vi "FM Voice Receiver - FIR.vi"() -> ()   [LabVIEW 2013]
uses:
  <vilib>/sound2/lvsound2.llb/Sound Output Write (DBL).vi
  <instrlib>/niUSRP/niUSRP Fetch Rx Data (CDB WDT).vi
  <vilib>/Analysis/3filter.llb/FIR Filter (DBL).vi
  <vilib>/Analysis/2dsp.llb/Rational Resample (single channel, DBL).vi
  <vilib>/express/express analysis/Spectral/Block/exnSpectralBlock spectral measurements RMS poly.vi
  <vilib>/express/express analysis/Spectral/Block/exnSpectralBlock spectral measurements RMS WFM.vi
  <vilib>/express/express analysis/Spectral/XNode/ExpressSpectralMeasurementsBlockNode.xnode
  <vilib>/Analysis/NI_AALPro.lvlib
  <vilib>/Analysis/NI_AALBase.lvlib
panel:
  out "File Error Out":errorcluster
  in  "Sound Format":T1={"sample rate (S/s)"=44100.0, "number of channels"=1.0, "bits per sample"=16.0}
  out "Spectrum (FFT)":cluster{"f0":dbl, "df":dbl, "magnitude":dbl[]}(graph)
  out "Waveform":waveform(dbl)(graph)
  out "Constellation":cluster{dbl[], dbl[]}(graph)
  out "USRP Error Out":errorcluster
  out "Coerced Gain":dbl format="%#_6f"
  out "Coerced Carrier Freq.":dbl=2400010000.007024 format="%#_6p"
  out "Coerced IQ Rate":dbl=200000.0 format="%#_6p"
  in  "Stop":bool
  in  "Active Antenna":string="RX2"
  in  "Gain":dbl format="%#_6f"
  in  "Carrier Frequency":dbl=1200000000.0 format="%#_6p"
  in  "IQ Rate":dbl=200000.0 format="%#_6p"
  in  "Device Address":refnum<k15>="192.168.10.2"
  in  "Number of Samples":i32=44100
  # "FM Receiver"
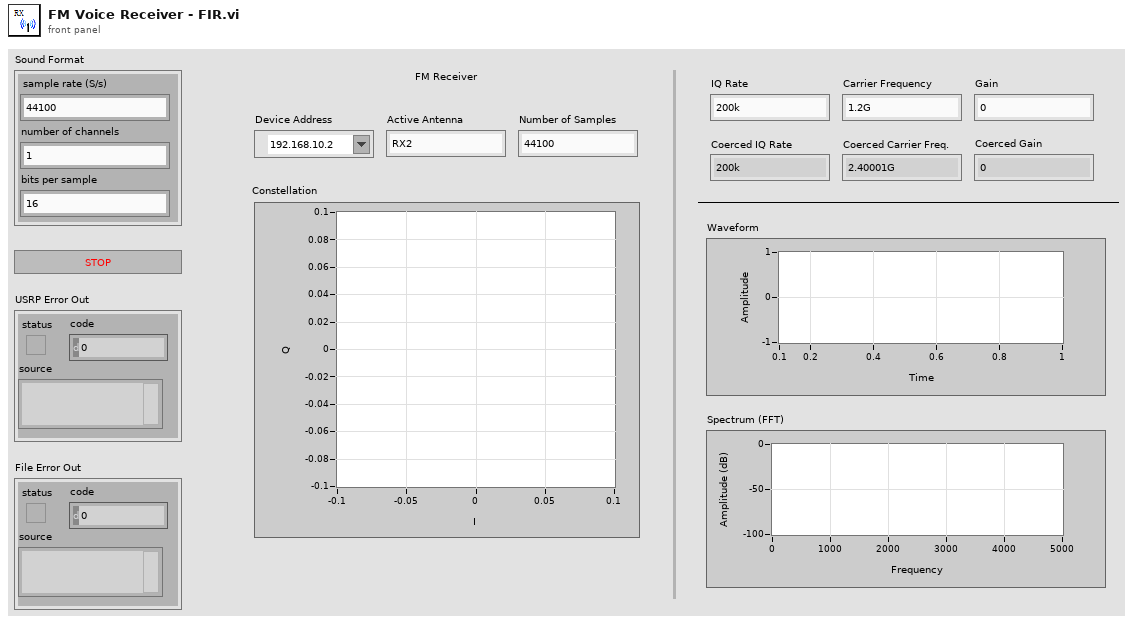
[diagram p1: front panel]
types:
  T1 = cluster{"sample rate (S/s)":dbl, "number of channels":dbl, "bits per sample":dbl}
  T2 = typedef "Sound Output Task ID.ctl" = u32
  T3 = cluster{"averaging mode":u16, "weighting mode":u16, "number of averages":u32}
  T4 = cluster{"dB On (F)":bool, "unwrap phase (F)":bool, "convert to degree (F)":bool}
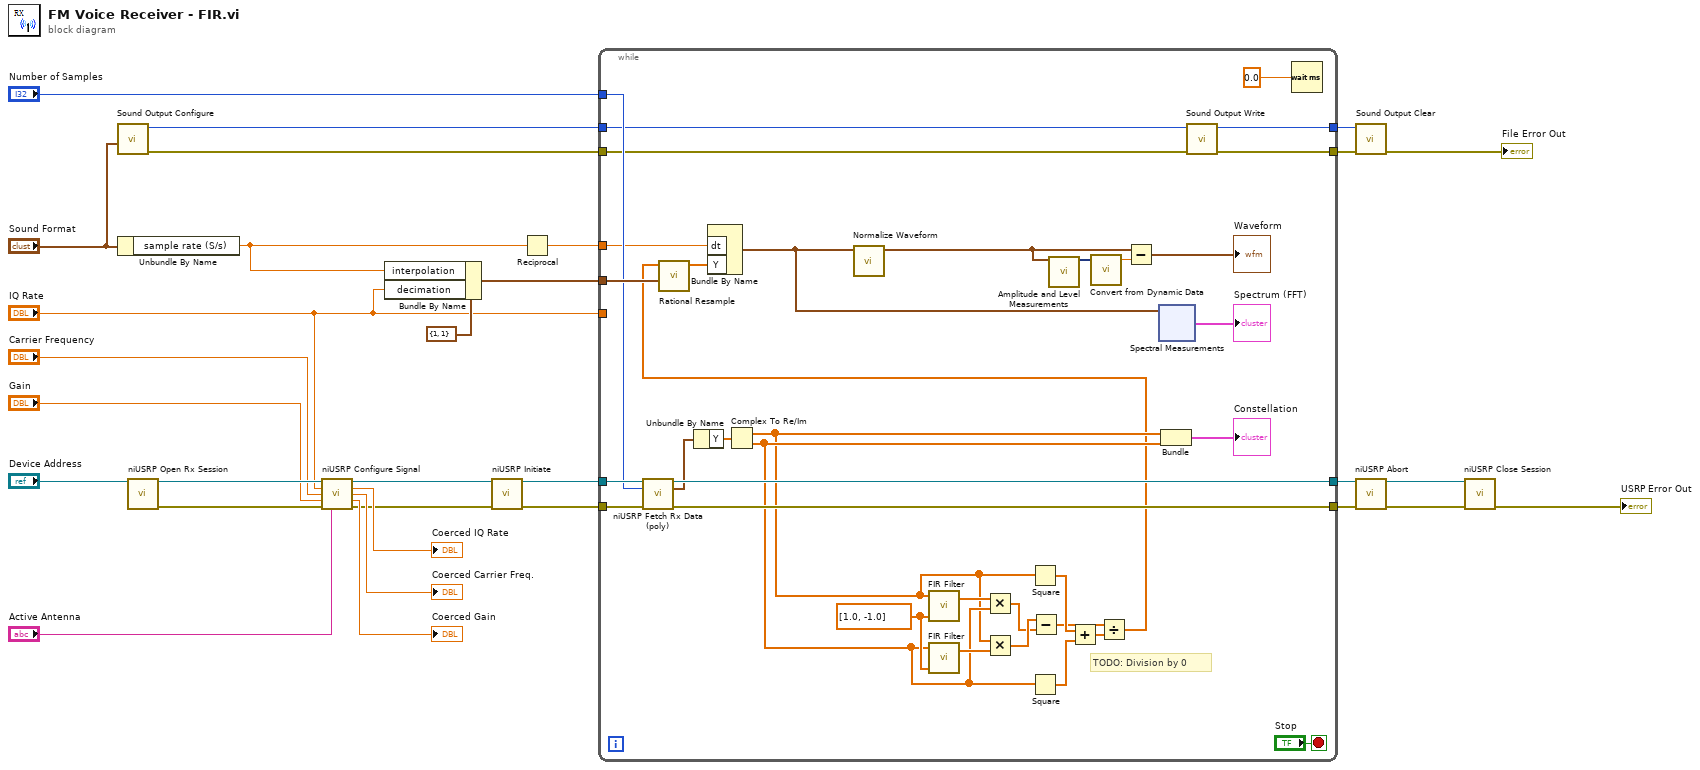
[diagram p0: block diagram]
diagram:
  n1 = call <vilib>:"Sound Output Configure.vi"("sound format"="Sound Format") -> ("error out"=w4:errorcluster, "task ID"=w5:T2)  [unwired: 9 in]
  n2 = Unbundle By Name("Sound Format") -> ("sample rate (S/s)"=w12:dbl)
  n3 = call <instrlib>:"niUSRP Open Rx Session.vi"("device names"="Device Address") -> ("session handle out"=w30:refnum<k15>, "error out"=w29:errorcluster)  [unwired: 13 in]
  n4 = call <instrlib>:"niUSRP Configure Signal.vi"("session handle"=w30, "IQ rate"="IQ Rate", "carrier frequency"="Carrier Frequency", "gain"="Gain", "error in (no error)"=w29, "active antenna"="Active Antenna") -> ("session handle out"=w16:refnum<k15>, "coerced IQ rate"=→"Coerced IQ Rate":dbl, "coerced carrier frequency"=→"Coerced Carrier Freq.":dbl, "coerced gain"=→"Coerced Gain":dbl, "error out"=w14:errorcluster)  [unwired: 5 in]
  n5 = Bundle By Name(cluster=cluster{"decimation":i32, "interpolation":i32} {"decimation"=1, "interpolation"=1}, "interpolation"=w12, "decimation"="IQ Rate") -> (w24:cluster{"decimation":i32, "interpolation":i32})
  n6 = call <instrlib>:"niUSRP Initiate.vi"("session handle"=w16, "error in (no error)"=w14) -> ("session handle out"=w15:refnum<k15>, "error out"=w13:errorcluster)  [unwired: 12 in]
  n7 = Reciprocal(x=w12) -> (1/x=w7:dbl)
  n8 = while {
    tunnel: w15 -> [w65]
    tunnel: [w63] -> w11
    tunnel: [w62] -> w10
    tunnel: w13 -> [w61]
    tunnel: "Number of Samples" -> [w57]
    tunnel: w24 -> [w60]
    tunnel: "IQ Rate" -> [_]
    tunnel: w7 -> [w53]
    tunnel: w5 -> [w52]
    tunnel: w4 -> [w51]
    tunnel: [w50] -> w3
    tunnel: [w49] -> w2
    stop <- "Stop" stop-if-true
    w38 = dbl[] [1.0, -1.0]
    # "TODO: Division by 0"
    n9 = call-poly <instrlib>:"niUSRP Fetch Rx Data (poly).vi"("session handle"=w65, "number of samples"=w57, "error in (no error)"=w61) -> ("session handle out"=w63:refnum<k15>, "data"=w43:waveform(cdb), "error out"=w62:errorcluster)  [unwired: 9 in, 1 out]
    n10 = Unbundle By Name(w43) -> ("Y"=w56:cdb[])
    n11 = Complex To Re/Im(x + iy=w56) -> (x=w36:dbl[], y=w37:dbl[])
    n12 = call-poly <vilib>:"FIR Filter.vi"("FIR Coefficients"=w38, "X"=w36) -> ("Filtered X"=w42:dbl[])  [unwired: 2 in, 1 out]
    n13 = call-poly <vilib>:"FIR Filter.vi"("FIR Coefficients"=w38, "X"=w37) -> ("Filtered X"=w41:dbl[])  [unwired: 2 in, 1 out]
    n14 = Multiply(x=w42, y=w37) -> (x*y=w39:dbl[])
    n15 = Multiply(x=w36, y=w41) -> (x*y=w40:dbl[])
    n16 = Square(x=w36) -> (x^2=w35:dbl[])
    n17 = Square(x=w37) -> (x^2=w34:dbl[])
    n18 = Subtract(x=w40, y=w39) -> (x-y=w33:dbl[])
    n19 = Add(x=w35, y=w34) -> (x+y=w32:dbl[])
    n20 = Divide(x=w33, y=w32) -> (x/y=w31:dbl[])
    n21 = call-poly <vilib>:"Rational Resample.vi"("resample factor"=w60, "X"=w31) -> ("Y"=w54:dbl[])  [unwired: 7 in, 2 out]
    n22 = Bundle By Name("dt"=w53, "Y"=w54) -> (w45:waveform(dbl))  [unwired: 1 in]
    n23 = call <vilib>:"Normalize Waveform.vi"("waveform in"=w45) -> ("normalized waveform"=w48:waveform(dbl))  [unwired: 7 in, 3 out]
    n24 = call "Amplitude and Level Measurements"("Signals"=w48) -> ("Mean (DC)"=w47:dynamicdata)  [unwired: 13 in, 1 out]
    n25 = call "Convert from Dynamic Data"("Dynamic Data Type"=w47) -> ("Scalar"=w46:dbl)  [unwired: 3 in]
    n26 = Subtract(x=w48, y=w46) -> (x-y=→"Waveform":waveform(dbl))
    n27 = xnode ("Spectral Measurements")("Signals"=w45) -> ("FFT - (RMS)"=→"Spectrum (FFT)":cluster{"f0":dbl, "df":dbl, "magnitude":dbl[]})  [unwired: 1 in, 2 out]
    n28 = Bundle(w36, w37) -> (→"Constellation":cluster{dbl[], dbl[]})  [unwired: 1 in]
    n29 = call-poly <vilib>:"Sound Output Write.vi"("error in (no error)"=w51, "task ID"=w52) -> ("error out"=w49:errorcluster, "task ID out"=w50:T2)  [unwired: 8 in]
    n30 = Wait (ms)(milliseconds to wait=0.0) -> ()  [unwired: 1 out]
  }
  n31 = call <vilib>:"Sound Output Clear.vi"("error in (no error)"=w2, "task ID"=w3) -> ("error out"=→"File Error Out":errorcluster)  [unwired: 9 in]
  n32 = call <instrlib>:"niUSRP Abort.vi"("session handle"=w11, "error in (no error)"=w10) -> ("session handle out"=w8:refnum<k15>, "error out"=w9:errorcluster)  [unwired: 12 in]
  n33 = call <instrlib>:"niUSRP Close Session.vi"("session handle"=w8, "error in (no error)"=w9) -> ("error out"=→"USRP Error Out":errorcluster)  [unwired: 13 in]
